vi "Configure Sweep Generation.vi"(5 "Auto Sweep or Dwell Time (T: Enable)":bool=TRUE, 6 "Sweep Generation (1: Analog)":i32(ring)=1 items=["Stepped", "Analog"], 7 "Sweep Points (201)":i32=201, 8 "error in (no error)":errorcluster, 9 "Sweep or Dwell Time (1 s)":dbl=1.0, 10 "Channel (1)":i32=1, 11 "VISA resource name":refnum<visa-resource-name>) -> (0 "error out":errorcluster, 3 "VISA resource name out":refnum<visa-resource-name>)   [LabVIEW 2018, in "Keysight PNA Series.lvlib"]
doc: "Configures the sweep generation."
uses:
  Keysight PNA Series.lvlib
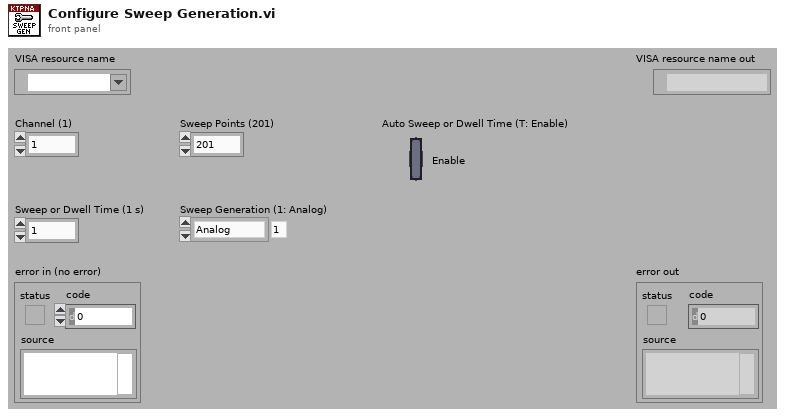
[diagram p1: front panel]
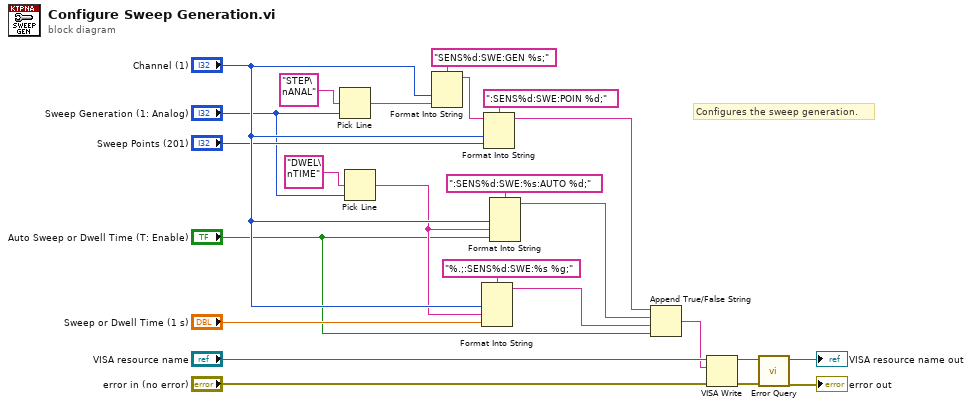
[diagram p0: block diagram]
diagram:
  # "Configures the sweep generation."
  n1 = Pick Line(multi-line string="STEP\nANAL", line index="Sweep Generation (1: Analog)") -> (output string=w21:string)  [unwired: 1 in]
  n2 = Pick Line(multi-line string="DWEL\nTIME", line index="Sweep Generation (1: Analog)") -> (output string=w7:string)  [unwired: 1 in]
  n3 = Format Into String(format string="SENS%d:SWE:GEN %s;", "Channel (1)", w21) -> (resulting string=w4:string)  [unwired: 2 in, 1 out]
  n4 = Format Into String(format string="%.;:SENS%d:SWE:%s %g;", "Channel (1)", w7, "Sweep or Dwell Time (1 s)") -> (resulting string=w5:string)  [unwired: 2 in, 1 out]
  n5 = Format Into String(format string=":SENS%d:SWE:POIN %d;", initial string=w4, "Channel (1)", "Sweep Points (201)") -> (resulting string=w2:string)  [unwired: 1 in, 1 out]
  n6 = Format Into String(format string=":SENS%d:SWE:%s:AUTO %d;", "Channel (1)", w7, "Auto Sweep or Dwell Time (T: Enable)") -> (resulting string=w6:string)  [unwired: 2 in, 1 out]
  n7 = Append True/False String(1:"Auto Sweep or Dwell Time (T: Enable)", 2:w5, 3:w6, 4:w2) -> (0:w1:string)
  n8 = VISA Write(VISA resource name="VISA resource name", write buffer=w1, error in (no error)="error in (no error)") -> (VISA resource name out=w14:refnum<visa-resource-name>, error out=w13:errorcluster)  [unwired: 1 out]
  n9 = call "Error Query.vi"("error in (no error)"=w13, "VISA resource name"=w14) -> ("error out"=→"error out":errorcluster, "VISA resource name out"=→"VISA resource name out":refnum<visa-resource-name>)  [unwired: 6 in, 2 out]
